vi "同步JK触发器.vi"(1 "k":bool, 2 "c":bool, 3 "J":bool) -> (0 "Q":bool)   [LabVIEW 2012, in "触发器.lvlib"]
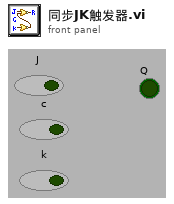
[diagram p1: front panel]
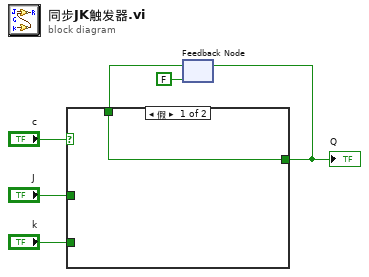
[diagram p0: block diagram]
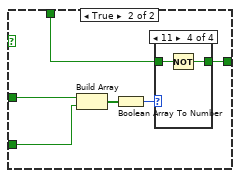
[diagram p2: hidden frame]
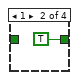
[diagram p4: hidden frame]
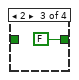
[diagram p5: hidden frame]
diagram:
  n1 = feedback #1(FALSE ("c")) -> (w5:bool)
  n2 = case shown="假" "c" {
    tunnel: w5 -> [w7 w13]
    tunnel: [w7 w12] -> w3
    tunnel: "J" -> [_ w10]
    tunnel: "k" -> [_ w9]
    frame False {
    }
    frame True {
      n3 = Build Array(w10, w9) -> (w11:bool[])
      n4 = Boolean Array To Number(Boolean array=w11) -> (number=w8:u32)
      n5 = case shown="11" w8 {
        tunnel: w13 -> [w14 _ _ w18]
        tunnel: [w14 TRUE ("c") FALSE ("c") w17] -> w12
        frame 0, Default {
        }
        frame 1 {
        }
        frame 2 {
        }
        frame 3 {
          n6 = Not(x=w18) -> (.not. x?=w17:bool)
        }
      }
    }
  }
  "Q" <- w3
  n7 = feedback-in #1(w3) -> ()
